vi "RT_main4.vi"() -> ()   [LabVIEW 2018]
uses:
  <vilib>/Platform/TimedLoop/XDataNode/timing_clust.ctl
  <vilib>/Platform/TimedLoop/XDataNode/nitl_modes.ctl
  <vilib>/Platform/TimedLoop/XDataNode/wakeup.ctl
  <vilib>/FPGAPlugInAG/myRIO-1900/niLvFpga_Open_myRIO-1900.vi
  <vilib>/rvi/interface/common/dynamic/niFpgaDynamicAddResources.vi
  <vilib>/Utility/error.llb/Error Cluster From Error Code.vi
  <vilib>/rvi/errors/niLvFpgaAdjustHostInterfaceError.vi
  <vilib>/addons/control/pid/pid.llb/PID (DBL).vi
  <vilib>/FPGAPlugInAG/Dynamic/niLvFpga_Close_Dynamic.vi
  <vilib>/rvi/interface/nirviOpenFPGA/nirviOpenFPGA.xnode
  FPGA Bitfiles/DQNcarpolelvsim_FPGATarget_FPGAsmall2_d4itNFSFwjs.lvbitx
  FPGA_small2.vi
  <vilib>/platform/TimedLoop/XDataNode/XDataNode.xnode
  <vilib>/rvi/interface/nirviReadWriteControl/nirviReadWriteControl.xnode
  <vilib>/rvi/interface/nirviCloseFPGA/nirviCloseFPGA.xnode
  <vilib>/rvi/interface/Simulation/niFpgaSimulationCallBeginRW.vi
  <vilib>/addons/control/pid/NI_PID_pid.lvlib
  NiFpgaLv.dll
  <vilib>/Platform/TimedLoop/XDataNode/XDNodeRunTimeDep.lvlib
panel:
  in  "speed st scale":dbl=0.8 format="%#_13g"
  in  "buf size":i32=16
  in  "s":bool
  in  "Period":i64=8
  in  "man":bool
  in  "Slide":i16(slide) scale=-500.0..500.0
  out "pos":T1(graph)={"Slide"=0, "set pt"=0, "position"=-1}
  out "dai Chart":cluster{"mean":dbl, dbl}(graph)
  in  "selctl":bool=TRUE
  out "set_pt":i16
  in  "scale":dbl=30.0
  out "pid output":u16(graph)=23
  in  "dx_sim":dbl=0.1
  out "gap_pos":i16=1
  out "states":dbl[](array[numeric])=[-1.0, 0.0, -1.438260386721577, 0.0]
  out "busy":bool
  out "off_track":bool
  out "output":u16=23
  in  "output range":cluster{"output high":dbl, "output low":dbl}={"output high"=80.0, "output low"=23.0} {"output low" format="%.2f"; "output high" format="%.2f"}
  out "dt (s)":dbl=0.008 format="%.3f"
  in  "PID gains":T2={"proportional gain (Kc)"=0.2, "integral time (Ti, min)"=0.0, "derivative time (Td, min)"=0.0006000000000000001} {"derivative time (Td, min)" format="%.5f"; "integral time (Ti, min)" format="%.5f"; "proportional gain (Kc)" format="%.4f"}
  out "speed Chart":i16(graph)
  out "position":i16=1
  in  "stop":bool
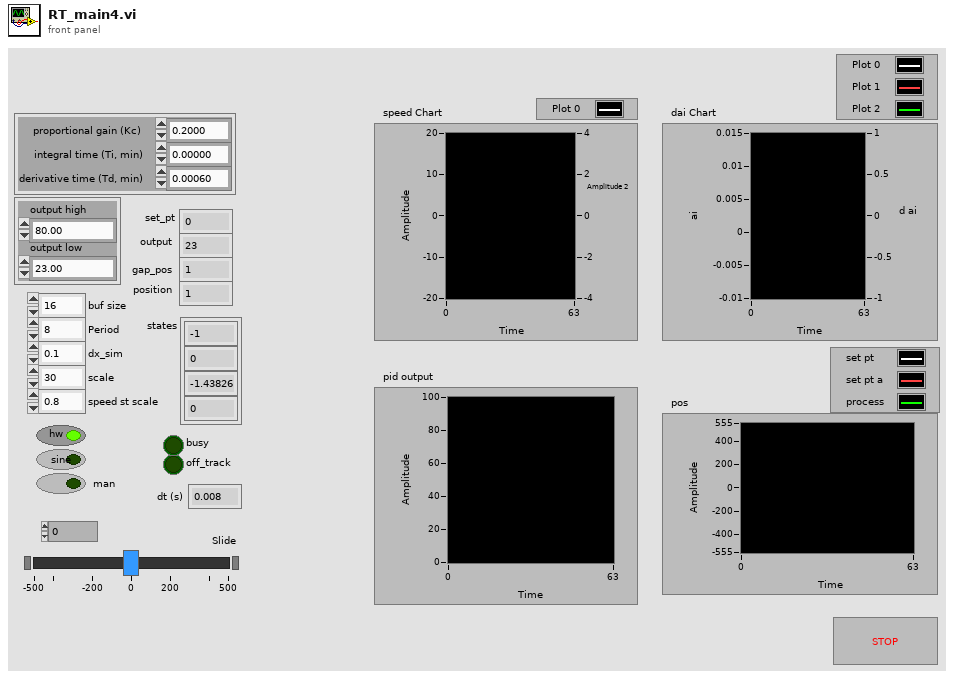
[diagram p1: front panel]
types:
  T1 = cluster{"Slide":i16, "set pt":i16, "position":i16}
  T2 = cluster{"proportional gain (Kc)":dbl, "integral time (Ti, min)":dbl, "derivative time (Td, min)":dbl}
  T3 = typedef "XDNodeRunTimeDep.lvlib/timing_clust.ctl" = cluster{"Expected End [f-1]":u64, "Actual End [f-1]":u64, "Finished Late? [f-1]":bool, "Expected End [i-1]":u64, "Actual End [i-1]":u64, "Finished Late? [i-1]":bool, "Expected Start [i]":u64, "Actual Start [i]":u64, "Expected Start [f]":u64, "Actual Start [f]":u64, "Source Name":string, "Structure Name":string, "Period":i64, "Deadline":i64, "Offset":i64, "Start":i64, "Priority":i32, "Timeout":i32, "Mode":T4, "Wakeup Reason":T5, "Error":errorcluster, "Source Type":string, "Secondary Source Type":string, "Global End Time":u64, "Global Start Time":u64, "Frame Duration":u64, "Iteration Duration":u64, "Assigned CPU":i32, "I/O Scan Engine Mode":u32}
  T4 = typedef "XDNodeRunTimeDep.lvlib/nitl_modes.ctl" = enum32{"No Change", "Process missed periods, maintain original phase", "Discard missed periods, maintain original phase", "Process missed periods, ignore original phase", "Discard missed periods, ignore original phase"}
  T5 = typedef "XDNodeRunTimeDep.lvlib/wakeup.ctl" = enum32{"Normal", "Aborted", "Asynchronous wakeup", "Timing source error", "Timed loop error", "Timeout"}
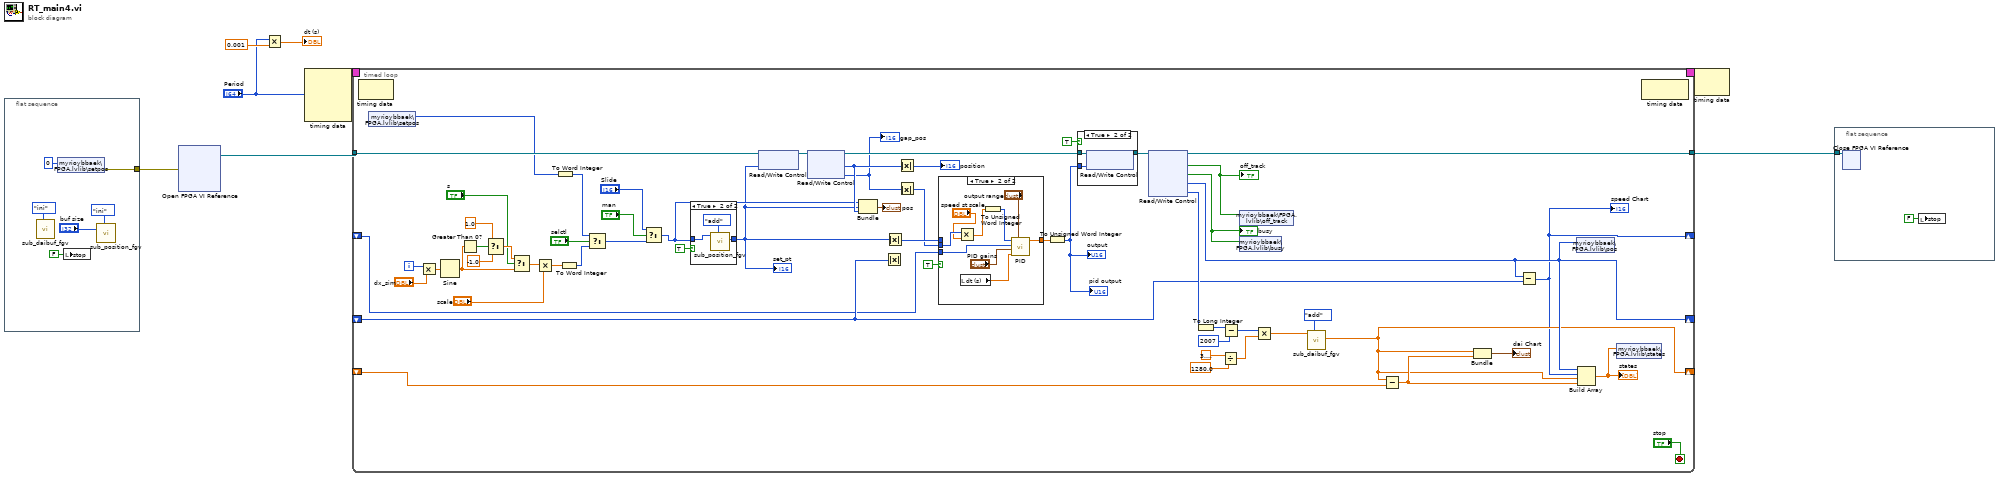
[diagram p0: block diagram]
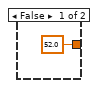
[diagram p4: hidden frame]
diagram:
  n1 = flat-sequence {
    tunnel: [w13] -> w2
    frame #0 {
      n2 = call "sub_daibuf_fgv.vi"("cmd"=enum16{"ini", "add"}."ini") -> ()  [unwired: 9 in, 2 out]
      n3 = shared-variable "myrioybbaek\\FPGA.lvlib\\setpos"(i16 0 ("setpos")) -> (error out=w13:errorcluster)  [unwired: 1 in]
      n4 = local write "stop"(FALSE ("stop")) -> ()
      n5 = call "sub_position_fgv.vi"("cmd"=enum16{"ini", "add"}."ini", "buf size"="buf size") -> ()  [unwired: 8 in, 2 out]
    }
  }
  n6 = xnode "Open FPGA VI Reference"("error in"=w2) -> ("FPGA VI Reference Out"=w1:refnum<k20>)  [unwired: 1 in, 1 out]
  n7 = Multiply(x="Period", y=0.001 ("t")) -> (x*y=→"dt (s)":dbl)
  n8 = node-c288("Period") -> (w5:T3)  [unwired: 3 in]
  n9 = timed-loop {
    tunnel: w1 -> [w72]
    tunnel: [w67] -> w8
    shift-right: [w19] -> _
    shift-left: _ -> [w47]
    shift-right: [w46] -> _
    shift-left: _ -> [w24]
    timing: w5 -> [_]
    timing-out: [_] -> w4
    shift-right: [w17] -> _
    shift-left: _ -> [w23]
    i -> [w55]
    stop <- "stop" stop-if-true
    n10 = node-c288() -> ()  [unwired: 1 in, 1 out]
    n11 = shared-variable "myrioybbaek\\FPGA.lvlib\\setpos"() -> (w25:i16)  [unwired: 1 in, 1 out]
    n12 = Multiply(x=w55, y="dx_sim") -> (x*y=w53:dbl)
    n13 = Sine(x=w53) -> (sin(x)=w28:dbl)
    n14 = Greater Than 0?(x=w28) -> (x > 0?=w37:bool)
    n15 = Select(t=1.0, s=w37, f=-1.0 ("t")) -> (s? t:f=w30:dbl)
    n16 = Select(t=w30, s="s", f=w28) -> (s? t:f=w29:dbl)
    n17 = Multiply(x=w29, y="scale") -> (x*y=w51:dbl)
    n18 = To Word Integer(number=w25) -> (16bit integer=w48:i16)
    n19 = To Word Integer(number=w51) -> (16bit integer=w49:i16)
    n20 = Select(t=w48, s="selctl", f=w49) -> (s? t:f=w41:i16)
    n21 = Select(t="Slide", s="man", f=w41) -> (s? t:f=w16:i16)
    n22 = case shown="True" TRUE {
      tunnel: w16 -> [w79 w81]
      tunnel: [w79 w80] -> w15
      frame False {
      }
      frame True {
        n23 = call "sub_position_fgv.vi"("cmd"=enum16{"ini", "add"}."add", "data"=w81) -> ("set pt"=w80:i16)  [unwired: 8 in, 1 out]
      }
    }
    "set_pt" <- w15
    n24 = xnode "Read/Write Control"("FPGA VI Reference In"=w72, "set_point"=w15) -> ("FPGA VI Reference Out"=w70:refnum<k20>)  [unwired: 1 in, 1 out]
    n25 = xnode "Read/Write Control"("FPGA VI Reference In"=w70) -> ("FPGA VI Reference Out"=w69:refnum<k20>, "position"=w39:i16, "gap_pos"=w32:i16)  [unwired: 1 in, 1 out]
    "gap_pos" <- w32
    n26 = Bundle("Slide"=w16, "set pt"=w15, "position"=w39) -> (→"pos":T1)  [unwired: 1 in]
    n27 = Absolute Value(x=w24) -> ()  [unwired: 1 out]
    n28 = Absolute Value(x=w15) -> (abs(x)=w34:i16)
    n29 = Absolute Value(x=w39) -> (abs(x)=→"position":i16)
    n30 = Absolute Value(x=w32) -> (abs(x)=w31:i16)
    n31 = case shown="True" TRUE {
      tunnel: [52.0 ("output") w90] -> w50
      tunnel: w34 -> [_ _]
      tunnel: w31 -> [_ w87]
      tunnel: w23 -> [_ w88]
      frame False {
      }
      frame True {
        n32 = Multiply(x=w87, y="speed st scale") -> (x*y=w85:dbl)
        n33 = local read "dt (s)"() -> (w89:dbl)
        n34 = To Unsigned Word Integer(number=w85) -> (unsigned 16bit integer=w84:u16)
        n35 = call-poly <vilib>:"PID.vi"("output range"="output range", "dt (s)"=w89, "PID gains"="PID gains", "process variable"=w88, "setpoint"=w84) -> ("output"=w90:dbl)  [unwired: 5 in, 1 out]
      }
    }
    n36 = To Unsigned Word Integer(number=w50) -> (unsigned 16bit integer=w43:u16)
    "output" <- w43
    "pid output" <- w43
    n37 = case shown="True" TRUE {
      tunnel: w69 -> [w73 w76]
      tunnel: [w73 w75] -> w68
      tunnel: w43 -> [_ w74]
      frame False {
      }
      frame True {
        n38 = xnode "Read/Write Control"("FPGA VI Reference In"=w76, "dt_pwm_us"=w74) -> ("FPGA VI Reference Out"=w75:refnum<k20>)  [unwired: 1 in, 1 out]
      }
    }
    n39 = xnode "Read/Write Control"("FPGA VI Reference In"=w68) -> ("FPGA VI Reference Out"=w67:refnum<k20>, "off_track"=w65:bool, "busy"=w57:bool, "position"=w46:i16, "AI0"=w56:u16)  [unwired: 1 in, 1 out]
    "off_track" <- w65
    "busy" <- w57
    n40 = To Long Integer(number=w56) -> (32bit integer=w64:i32)
    n41 = Divide(x=3.141592653589793, y=1280.0) -> (x/y=w63:dbl)
    n42 = Subtract(x=w64, y=u16 2007) -> (x-y=w62:i32)
    n43 = shared-variable "myrioybbaek\\FPGA.lvlib\\off_track"(w65) -> ()  [unwired: 1 in, 1 out]
    n44 = shared-variable "myrioybbaek\\FPGA.lvlib\\busy"(w57) -> ()  [unwired: 1 in, 1 out]
    n45 = Multiply(x=w62, y=w63) -> (x*y=w20:dbl)
    n46 = call "sub_daibuf_fgv.vi"("cmd"=enum16{"ini", "add"}."add", "data"=w20) -> ("mean"=w19:dbl)  [unwired: 8 in, 1 out]
    n47 = Subtract(x=w19, y=w47) -> (x-y=w21:dbl)
    n48 = Bundle("mean"=w19, w21) -> (→"dai Chart":cluster{"mean":dbl, dbl})  [unwired: 1 in]
    n49 = Subtract(x=w46, y=w24) -> (x-y=w17:i16)
    "speed Chart" <- w17
    n50 = shared-variable "myrioybbaek\\FPGA.lvlib\\pos"(w46) -> ()  [unwired: 1 in, 1 out]
    n51 = Build Array(w46, w17, w19, w21) -> (w58:dbl[])
    "states" <- w58
    n52 = shared-variable "myrioybbaek\\FPGA.lvlib\\states"(w58) -> ()  [unwired: 1 in, 1 out]
    n53 = node-c288() -> ()  [unwired: 1 in, 1 out]
  }
  n54 = node-c288(w4) -> ()  [unwired: 1 out]
  n55 = flat-sequence {
    tunnel: w8 -> [w94]
    frame #0 {
      n56 = xnode "Close FPGA VI Reference"("FPGA VI Reference In"=w94) -> ()  [unwired: 1 in, 1 out]
      n57 = local write "stop"(FALSE ("stop")) -> ()
    }
  }
